vi "Temp_Coeff_Read.vi"(8 "error in (no error)":errorcluster, 11 "BMP208 in":refnum<class "BMP208.lvclass">) -> (0 "error out":errorcluster, 3 "BMP208 out":refnum<class "BMP208.lvclass">)   [LabVIEW 2020, in "BMP208.lvclass"]
uses:
  BMP208.lvclass
  Controls/td_cluster_Temp_Coeff.ctl
  BMP208.lvclass/BMP208.ctl
  Write TempCoeff.vi
  LINX I2C/LINX I2C.lvclass
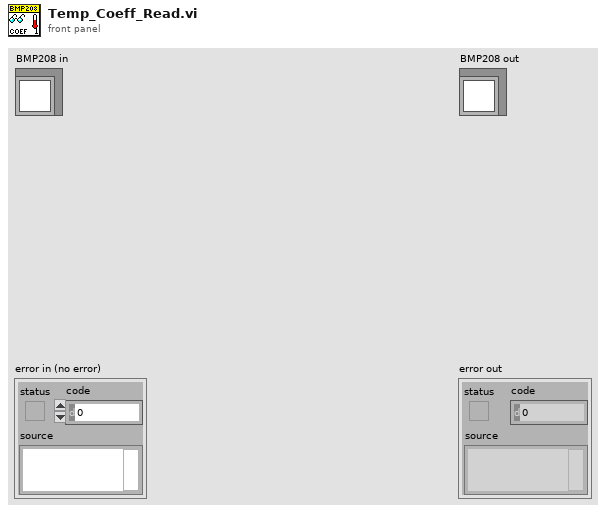
[diagram p1: front panel]
types:
  T1 = typedef "BMP208.lvclass/td_cluster_Temp_Coeff.ctl" = cluster{"T1":u16, "T2":i16, "T3":i16}
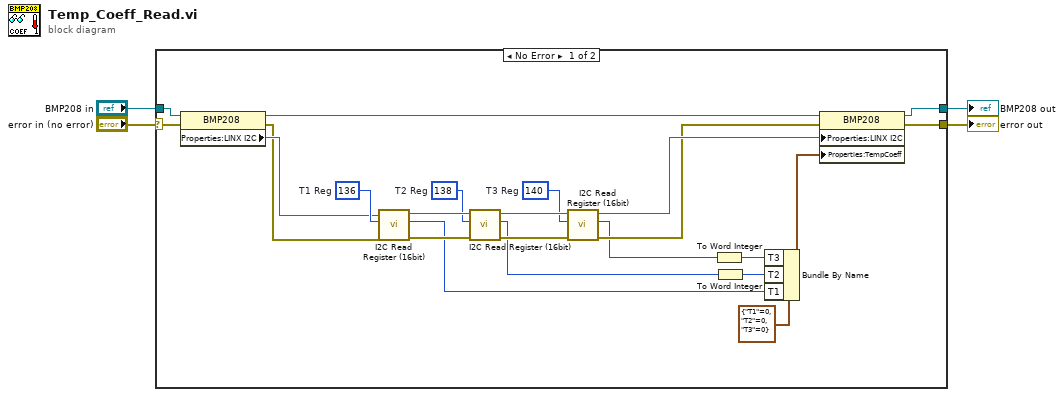
[diagram p0: block diagram]
diagram:
  n1 = case shown="No Error" "error in (no error)" {
    selector: "error in (no error)" -> [w27 w29]
    tunnel: [w25 w29] -> w3
    tunnel: [w23 w28] -> w1
    tunnel: "BMP208 in" -> [w26 w28]
    frame No Error {
      w16 = u8 140  # T3 Reg
      w17 = u8 138  # T2 Reg
      w22 = u8 136  # T1 Reg
      n2 = property class="BMP208"(reference=w26, error in=w27) -> (reference out=w24:refnum<class "BMP208.lvclass">, error out=w13:errorcluster, "Properties:LINX I2C"=w14:refnum<class "LINX I2C.lvclass">)
      n3 = call "I2C Read Register (16bit).vi"("error in (no error)"=w13, "Register Address"=w22, "LINX I2C in"=w14) -> ("error out"=w20:errorcluster, "Value"=w7:u16, "LINX I2C out"=w21:refnum<class "LINX I2C.lvclass">)  [unwired: 6 in]
      n4 = call "I2C Read Register (16bit).vi"("error in (no error)"=w20, "Register Address"=w17, "LINX I2C in"=w21) -> ("error out"=w18:errorcluster, "Value"=w8:u16, "LINX I2C out"=w19:refnum<class "LINX I2C.lvclass">)  [unwired: 6 in]
      n5 = call "I2C Read Register (16bit).vi"("error in (no error)"=w18, "Register Address"=w16, "LINX I2C in"=w19) -> ("error out"=w12:errorcluster, "Value"=w9:u16, "LINX I2C out"=w15:refnum<class "LINX I2C.lvclass">)  [unwired: 6 in]
      n6 = To Word Integer(number=w9) -> (16bit integer=w6:i16)
      n7 = To Word Integer(number=w8) -> (16bit integer=w5:i16)
      n8 = Bundle By Name(cluster=T1 {"T1"=0, "T2"=0, "T3"=0} ("TempCoeff"), "T3"=w6, "T2"=w5, "T1"=w7) -> (w10:T1)
      n9 = property class="BMP208"(reference=w24, error in=w12, "Properties:LINX I2C"=w15, "Properties:TempCoeff"=w10) -> (reference out=w23:refnum<class "BMP208.lvclass">, error out=w25:errorcluster)
    }
    frame Error {
    }
  }
  "error out" <- w3
  "BMP208 out" <- w1
